vi "version.vi"() -> ()   [LabVIEW 2011]
panel:
  in  "version":string
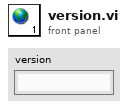
[diagram p1: front panel]
diagram:
